vi "Stop Subpanel UI.vi"(8 "error in (no error)":errorcluster, 11 "Controller in":refnum<class "Generic Plugin.lvclass">) -> (0 "error out":errorcluster, 3 "Controller out":refnum<class "Generic Plugin.lvclass">)   [LabVIEW 2020, in "Generic Plugin.lvclass"]
uses:
  Generic Plugin.lvclass
  Generic Plugin.lvclass/Generic Plugin.ctl
  Sub VIs/Message Queue/test Message Queue.lvlib
  Sub VIs/Message Queue/Enqueue Message (Single).vi
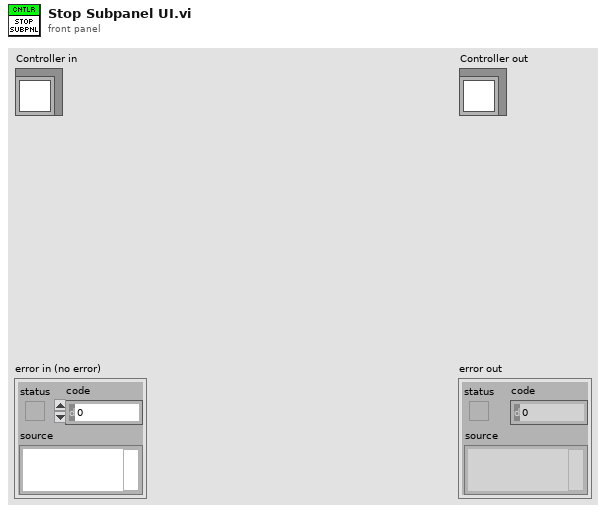
[diagram p1: front panel]
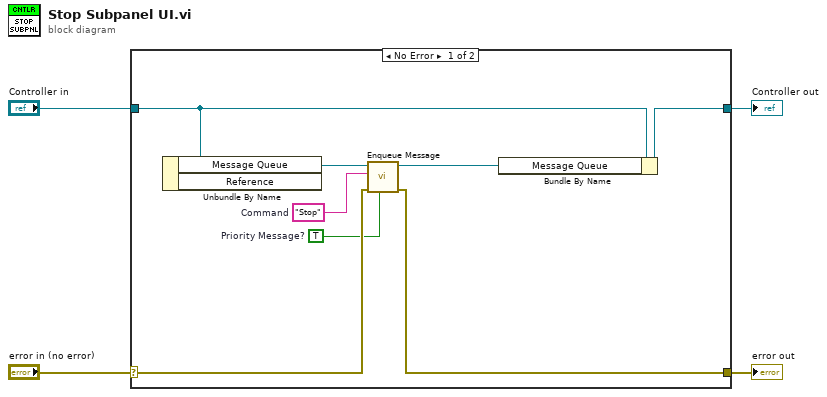
[diagram p0: block diagram]
diagram:
  n1 = case shown="No Error" "error in (no error)" {
    selector: "error in (no error)" -> [w7 w14]
    tunnel: [w5 w14] -> w3
    tunnel: [w9 w13] -> w1
    tunnel: "Controller in" -> [w12 w13]
    frame No Error {
      w6 = TRUE  # Priority Message?
      w10 = "Stop"  # Command
      n2 = Unbundle By Name(w12) -> ("Message Queue"=w11:refnum<queue>)  [unwired: 1 out]
      n3 = call-poly "Enqueue Message.vi"("Priority Message? (F)"=w6, "error in (no error)"=w7, "Message"=w10, "Message Queue"=w11) -> ("error out"=w5:errorcluster, "dup Message Queue"=w8:refnum<queue>)  [unwired: 6 in]
      n4 = Bundle By Name(cluster=w12, "Message Queue"=w8) -> (w9:refnum<class "Generic Plugin.lvclass">)
    }
    frame Error {
    }
  }
  "error out" <- w3
  "Controller out" <- w1
